vi "Build Profile Steps Commands.vi"(8 "error in":errorcluster, 11 "Profile Steps":string[][](array[string])) -> (0 "error out":errorcluster, 2 "Param Only Commands":T1[](array[typedef]), 3 "Profile Steps Commands":T1[](array[typedef]))   [LabVIEW 2018, in "F4T.lvlib" / "F4T.lvclass"]
doc: "This VI takes a 2D string array containing the temperature chamber profiles steps and outputs the corresponding commands needed for setting the profile to the temperature chamber."
uses:
  F4T.lvclass
  Custom Controls/Command Data.ctl
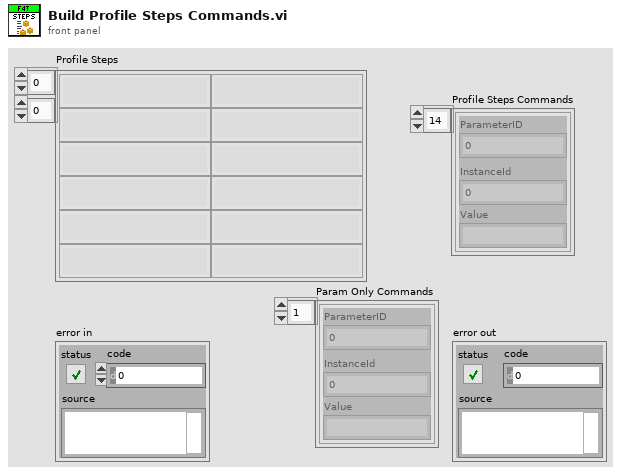
[diagram p1: front panel]
types:
  T1 = typedef "F4T.lvlib/F4T.lvclass/Command Data.ctl" = cluster{"ParameterID":u32, "InstanceId":u32, "Value":string}
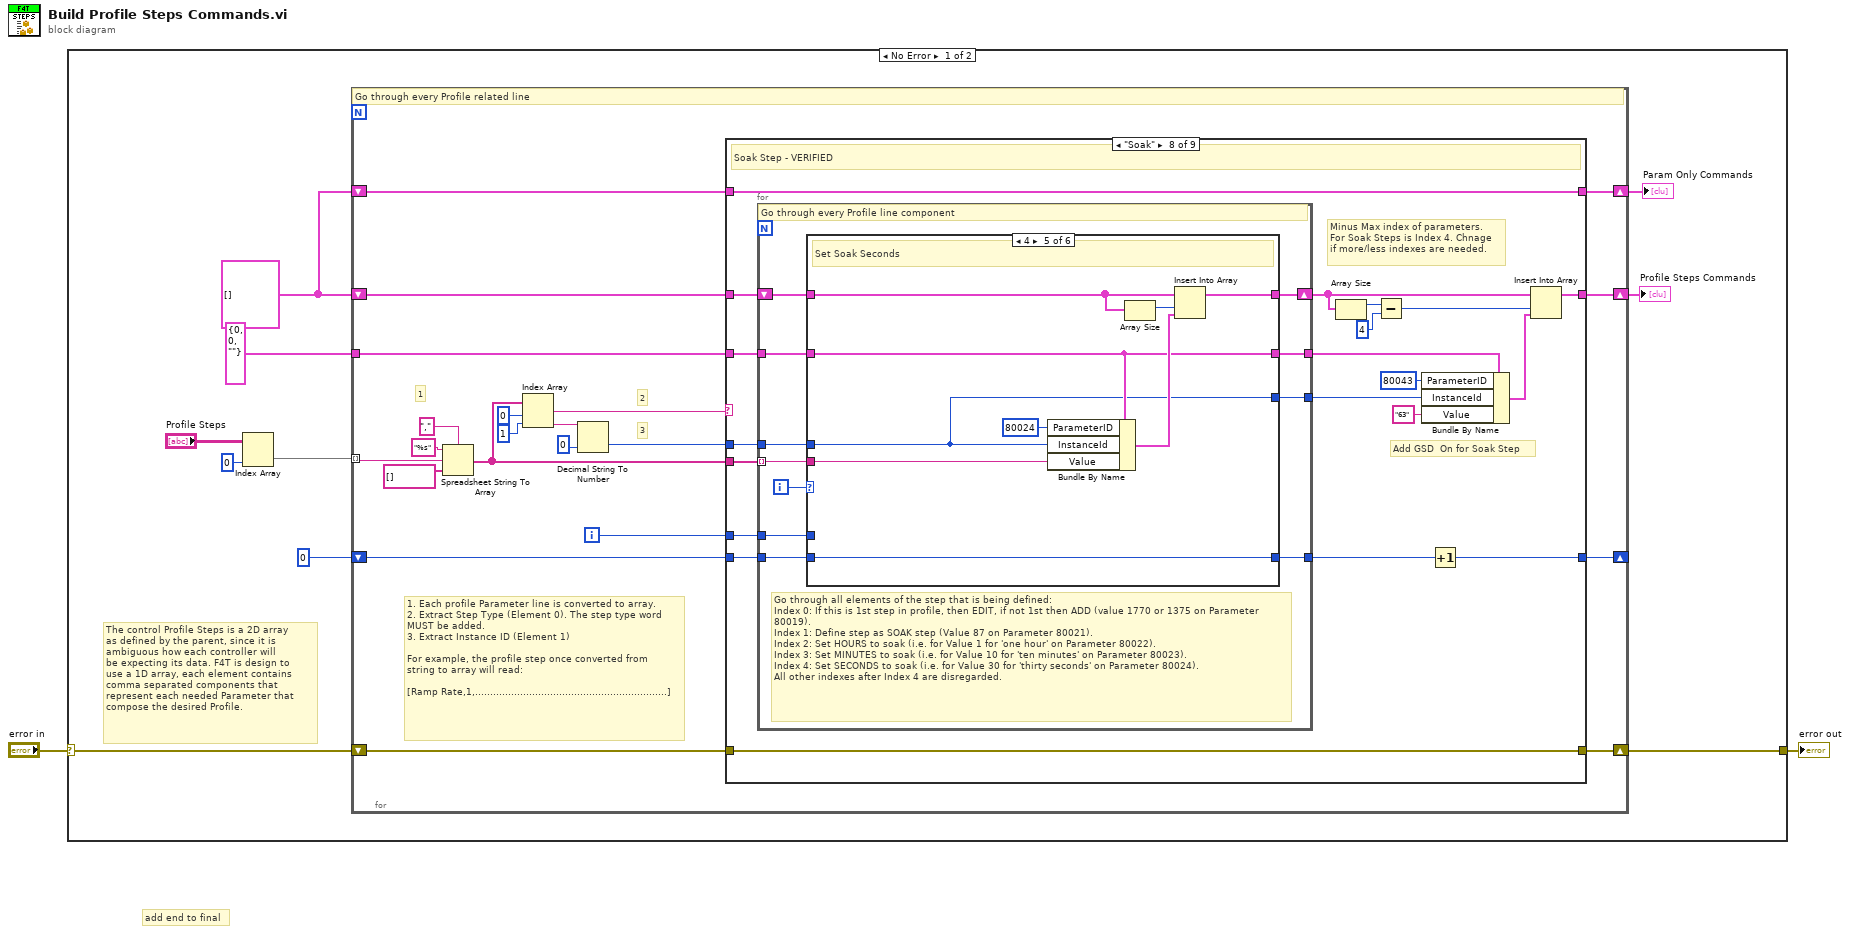
[diagram p0: block diagram]
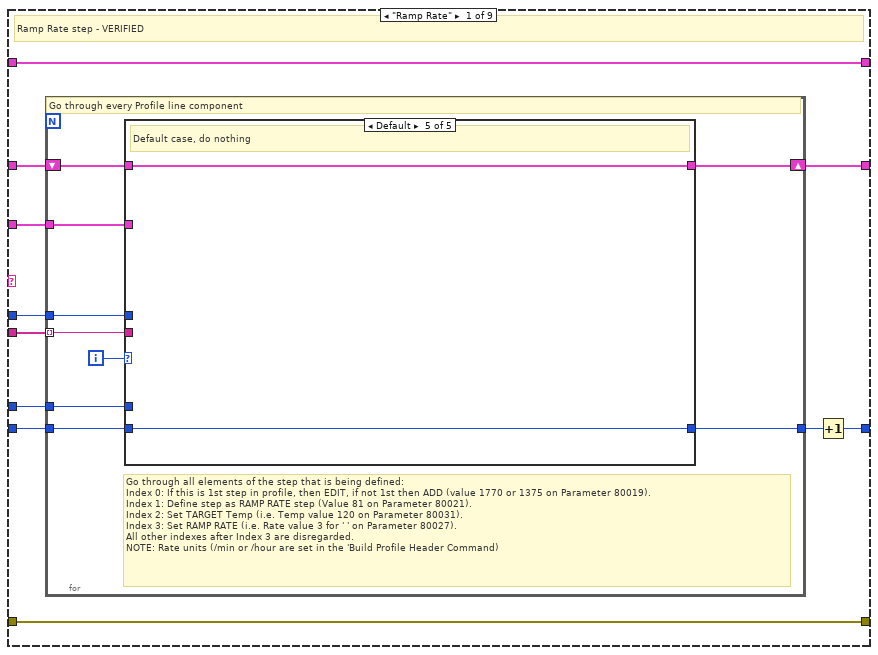
[diagram p2: hidden frame]
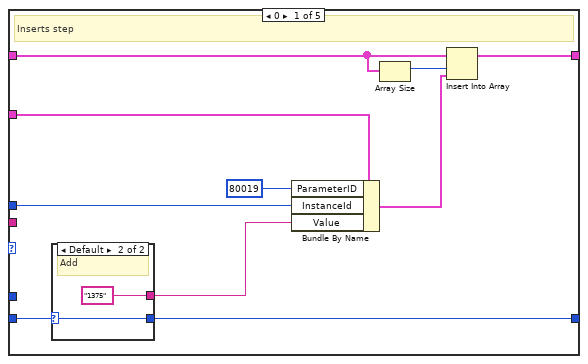
[diagram p3: hidden frame]
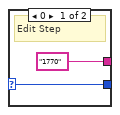
[diagram p4: hidden frame]
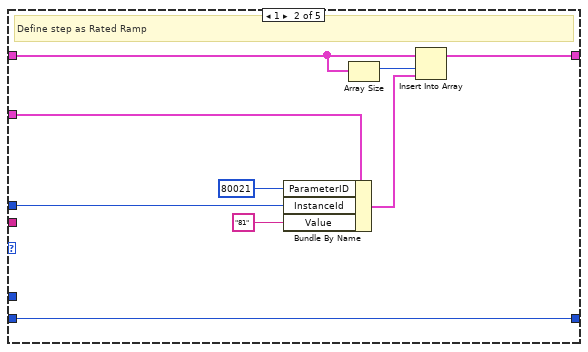
[diagram p5: hidden frame]
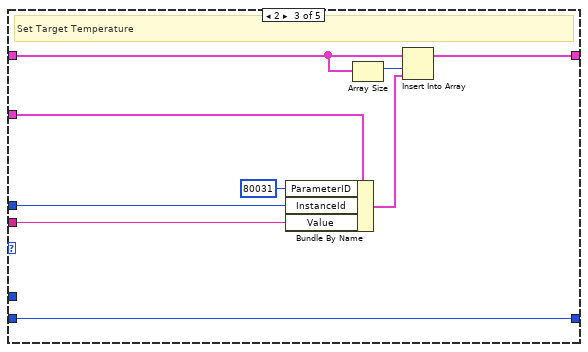
[diagram p6: hidden frame]
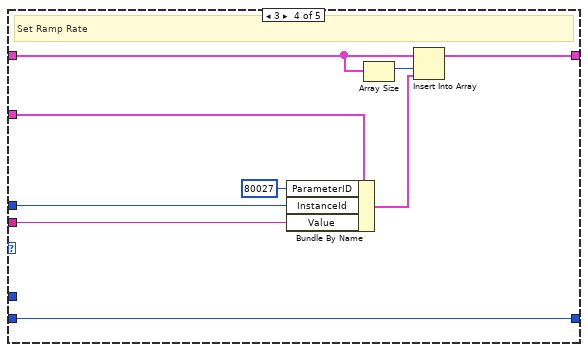
[diagram p7: hidden frame]
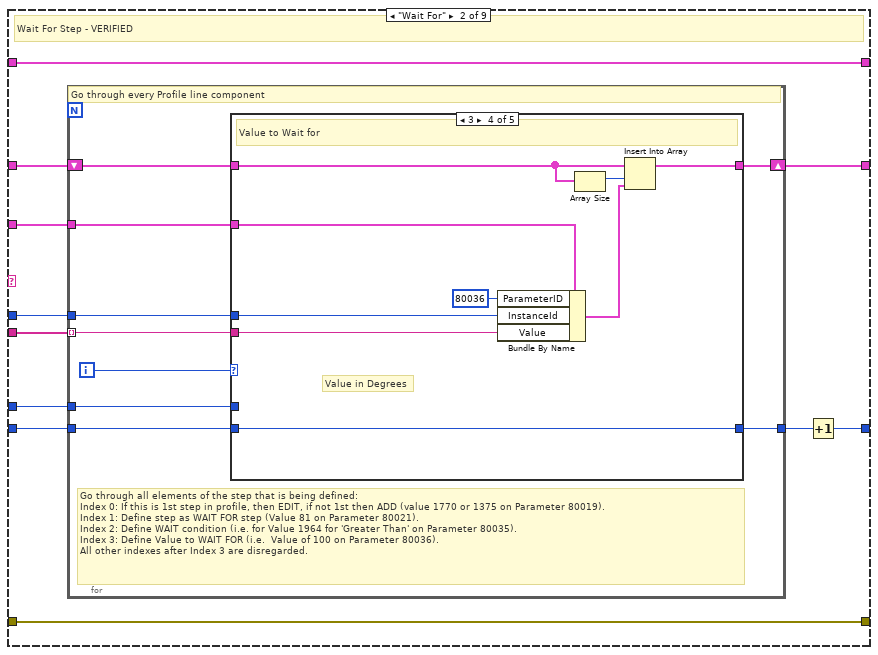
[diagram p8: hidden frame]
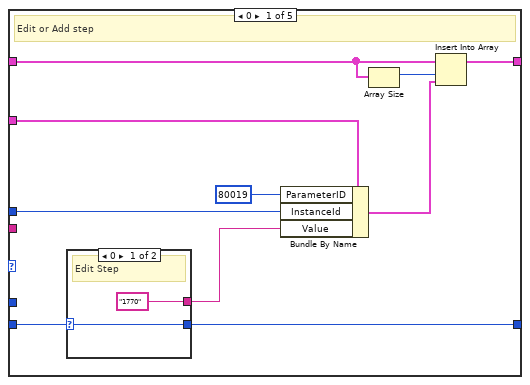
[diagram p9: hidden frame]
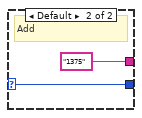
[diagram p10: hidden frame]
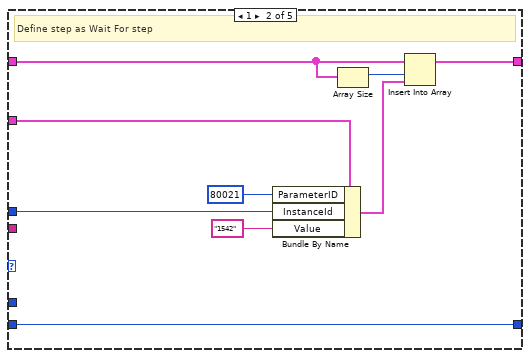
[diagram p11: hidden frame]
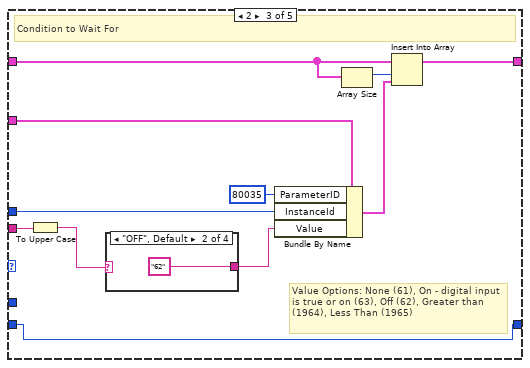
[diagram p12: hidden frame]
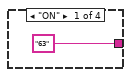
[diagram p13: hidden frame]
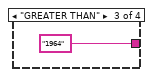
[diagram p14: hidden frame]
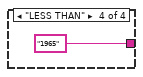
[diagram p15: hidden frame]
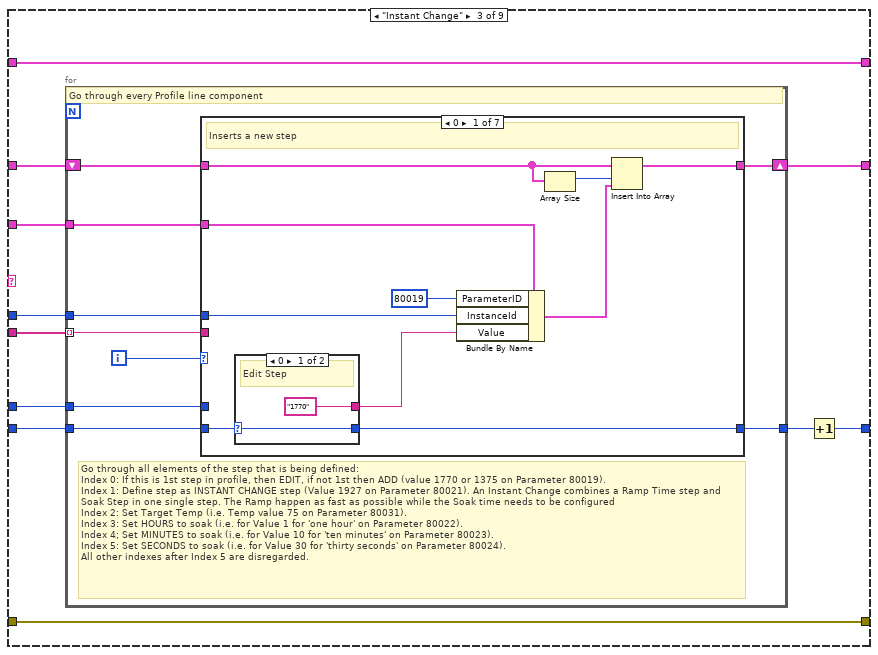
[diagram p17: hidden frame]
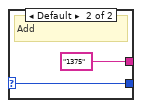
[diagram p18: hidden frame]
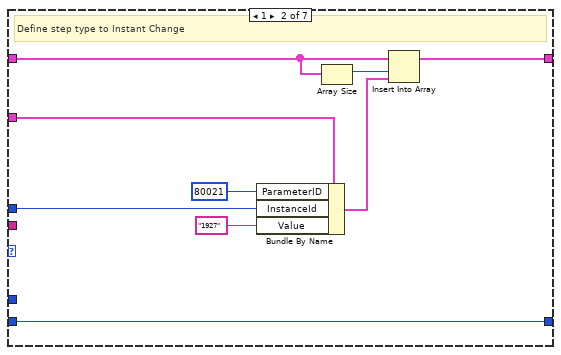
[diagram p19: hidden frame]
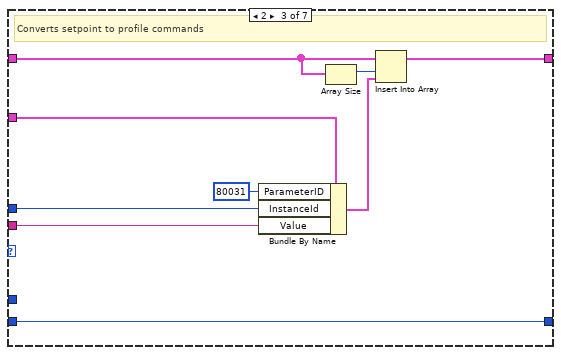
[diagram p20: hidden frame]
diagram:
  # "add end to final"
  n1 = case shown="No Error" "error in" {
    selector: "error in" -> [w11 w555]
    tunnel: [w10 w555] -> w1
    frame No Error {
      w5 = T1[] []
      # "The control Profile Steps is a 2D array\nas defined by the parent, since it is \nambiguous how each controller will\nbe expecting its data. F4T is design to\nuse a 1D array, each element contains\ncomma separated components that\nrepresent each needed Parameter that\ncompose the desired Profile."
      n2 = Index Array(array="Profile Steps", index (col)=0 ("disabled index (col)")) -> (element=w6:string[])  [unwired: 1 in]
      n3 = for {
        tunnel: w6 -> [w25] mode=indexing
        shift-right: [w19] -> w10
        shift-left: w11 -> [w18]
        shift-right: [w29] -> w12
        shift-left: w5 -> [w31]
        tunnel: T1 {"ParameterID"=0, "InstanceId"=0, "Value"=""} ("Command Data") -> [w30]
        shift-right: [w15] -> w4
        shift-left: w5 -> [w16]
        shift-right: [w13] -> _
        shift-left: 0 -> [w14]
        i -> [w17]
        # "3"
        # "1. Each profile Parameter line is converted to array. \n2. Extract Step Type (Element 0). The step type word\nMUST be added.\n3. Extract Instance ID (Element 1)\n\nFor example, the profile step once converted from\nstring to array will read:\n\n[Ramp Rate,1,................................................................]"
        # "1"
        # "2"
        # "Go through every Profile related line"
        n4 = Spreadsheet String To Array(delimiter (Tab)=",", format string="%s", spreadsheet string=w25, array type (2D Dbl)=string[] []) -> (array=w24:string[])
        n5 = Index Array(array=w24, index #1=0 ("index"), index #2=1 ("index")) -> (element #1=w32:string, element #2=w21:string)
        n6 = Decimal String To Number(string=w21, default (0L)=u32 0 ("default (0 I32)")) -> (number=w20:u32)  [unwired: 1 in, 1 out]
        n7 = case shown="\"Soak\"" w32 {
          tunnel: w24 -> [w43 w106 w175 w252 w322 w375 _ w469 w549]
          tunnel: w31 -> [w44 w107 w176 w257 w327 w376 w450 w470 w540]
          tunnel: w30 -> [w42 w105 w174 w256 w326 w374 _ w468 w554]
          tunnel: [w41 w104 w173 w255 w319 w373 w450 w464 w540] -> w29
          tunnel: w20 -> [w40 w103 w172 w253 w323 w372 _ w467 w550]
          tunnel: [w39 w102 w171 w254 w325 w371 w449 w466 w553] -> w19
          tunnel: w18 -> [w39 w102 w171 w254 w325 w371 w449 w466 w553]
          tunnel: w17 -> [w38 w101 w170 w251 w324 w370 _ w465 _]
          tunnel: w16 -> [w37 w100 w169 w250 w313 w369 w448 w454 w542]
          tunnel: [w37 w100 w169 w250 w313 w369 w448 w454 w541] -> w15
          tunnel: w14 -> [w36 w99 w168 w249 w312 w368 w447 w453 w537]
          tunnel: [w34 w97 w166 w247 w310 w366 w447 w451 w536] -> w13
          frame "Ramp Rate" {
            # "Ramp Rate step - VERIFIED"
            n8 = for {
              tunnel: w43 -> [w50] mode=indexing
              tunnel: w40 -> [w49]
              shift-right: [w53] -> w41
              shift-left: w44 -> [w51]
              tunnel: w42 -> [w48]
              tunnel: w38 -> [w47]
              tunnel: w36 -> [w46]
              tunnel: [w45] -> w35
              i -> [w52]
              # "Go through all elements of the step that is being defined:\nIndex 0: If this is 1st step in profile, then EDIT, if not 1st then ADD (value 1770 or 1375 on Parameter 80019).\nIndex 1: Define step as RAMP RATE step (Value 81 on Parameter 80021).\nIndex 2: Set TARGET Temp (i.e. Temp value 120 on Parameter 80031).\nIndex 3: Set RAMP RATE (i.e. Rate value 3 for ' ' on Parameter 80027).\nAll other indexes after Index 3 are disregarded.\nNOTE: Rate units (/min or /hour are set in the 'Build Profile Header Command)"
              # "Go through every Profile line component"
              n9 = case shown="Default" w52 {
                tunnel: [w59 w70 w85 w94 w96] -> w53
                tunnel: w51 -> [w58 w71 w84 w93 w96]
                tunnel: w50 -> [_ _ w81 w87 _]
                tunnel: w49 -> [w62 w74 w83 w92 _]
                tunnel: w48 -> [w60 w73 w82 w91 _]
                tunnel: w47 -> [_ _ _ _ _]
                tunnel: w46 -> [w55 w68 w77 w86 w95]
                tunnel: [w54 w68 w77 w86 w95] -> w45
                frame 0 {
                  # "Inserts step"
                  n10 = case shown="Default" w55 {
                    selector: w55 -> [w64 w66]
                    tunnel: ["1770" ("Value") "1375" ("Value")] -> w56
                    tunnel: [w64 w66] -> w54
                    frame 0 {
                      # "Edit Step"
                    }
                    frame Default {
                      # "Add"
                    }
                  }
                  n11 = Bundle By Name(cluster=w60, "ParameterID"=u32 80019, "InstanceId"=w62, "Value"=w56) -> (w57:T1)
                  n12 = Array Size(array=w58) -> (size(s)=w61:i32)
                  n13 = Insert Into Array(array=w58, index=w61, new element=w57) -> (w59:T1[])
                }
                frame 1 {
                  # "Define step as Rated Ramp"
                  n14 = Bundle By Name(cluster=w73, "ParameterID"=u32 80021, "InstanceId"=w74, "Value"="81") -> (w69:T1)
                  n15 = Array Size(array=w71) -> (size(s)=w72:i32)
                  n16 = Insert Into Array(array=w71, index=w72, new element=w69) -> (w70:T1[])
                }
                frame 2 {
                  # "Set Target Temperature"
                  n17 = Bundle By Name(cluster=w82, "ParameterID"=u32 80031, "InstanceId"=w83, "Value"=w81) -> (w78:T1)
                  n18 = Array Size(array=w84) -> (size(s)=w79:i32)
                  n19 = Insert Into Array(array=w84, index=w79, new element=w78) -> (w85:T1[])
                }
                frame 3 {
                  # "Set Ramp Rate"
                  n20 = Bundle By Name(cluster=w91, "ParameterID"=u32 80027, "InstanceId"=w92, "Value"=w87) -> (w88:T1)
                  n21 = Array Size(array=w93) -> (size(s)=w89:i32)
                  n22 = Insert Into Array(array=w93, index=w89, new element=w88) -> (w94:T1[])
                }
                frame Default {
                  # "Default case, do nothing"
                }
              }
            }
            n23 = Increment(x=w35) -> (x+1=w34:i32)
          }
          frame "Wait For" {
            # "Wait For Step - VERIFIED"
            n24 = for {
              tunnel: w106 -> [w113] mode=indexing
              tunnel: w103 -> [w112]
              shift-right: [w116] -> w104
              shift-left: w107 -> [w114]
              tunnel: w105 -> [w111]
              tunnel: w101 -> [w110]
              tunnel: w99 -> [w109]
              tunnel: [w108] -> w98
              i -> [w115]
              # "Go through all elements of the step that is being defined:\nIndex 0: If this is 1st step in profile, then EDIT, if not 1st then ADD (value 1770 or 1375 on Parameter 80019).\nIndex 1: Define step as WAIT FOR step (Value 81 on Parameter 80021).\nIndex 2: Define WAIT condition (i.e. for Value 1964 for 'Greater Than' on Parameter 80035).\nIndex 3: Define Value to WAIT FOR (i.e.  Value of 100 on Parameter 80036).\nAll other indexes after Index 3 are disregarded."
              # "Go through every Profile line component"
              n25 = case shown="3" w115 {
                tunnel: [w121 w133 w150 w163 w165] -> w116
                tunnel: w114 -> [w120 w134 w149 w162 w165]
                tunnel: w113 -> [_ _ w143 w156 _]
                tunnel: w112 -> [w124 w137 w148 w161 _]
                tunnel: w111 -> [w122 w136 w147 w160 _]
                tunnel: w110 -> [_ _ _ _ _]
                tunnel: w109 -> [w118 w131 w140 w155 w164]
                tunnel: [w117 w131 w140 w155 w164] -> w108
                frame 0 {
                  # "Edit or Add step"
                  n26 = case shown="0" w118 {
                    selector: w118 -> [w127 w129]
                    tunnel: ["1770" ("Value") "1375" ("Value")] -> w125
                    tunnel: [w127 w129] -> w117
                    frame 0 {
                      # "Edit Step"
                    }
                    frame Default {
                      # "Add"
                    }
                  }
                  n27 = Bundle By Name(cluster=w122, "ParameterID"=u32 80019, "InstanceId"=w124, "Value"=w125) -> (w119:T1)
                  n28 = Array Size(array=w120) -> (size(s)=w123:i32)
                  n29 = Insert Into Array(array=w120, index=w123, new element=w119) -> (w121:T1[])
                }
                frame 1 {
                  # "Define step as Wait For step"
                  n30 = Bundle By Name(cluster=w136, "ParameterID"=u32 80021, "InstanceId"=w137, "Value"="1542") -> (w132:T1)
                  n31 = Array Size(array=w134) -> (size(s)=w135:i32)
                  n32 = Insert Into Array(array=w134, index=w135, new element=w132) -> (w133:T1[])
                }
                frame 2 {
                  # "Value Options: None (61), On - digital input is true or on (63), Off (62), Greater than (1964), Less Than (1965)"
                  # "Condition to Wait For"
                  n33 = To Upper Case(1:w143) -> (0:w142:string)
                  n34 = case shown="\"OFF\", Default" w142 {
                    tunnel: ["63" ("Value") "62" ("Value") "1964" ("Value") "1965" ("Value")] -> w141
                    frame "ON" {
                    }
                    frame "OFF", Default {
                    }
                    frame "GREATER THAN" {
                    }
                    frame "LESS THAN" {
                    }
                  }
                  n35 = Bundle By Name(cluster=w147, "ParameterID"=u32 80035, "InstanceId"=w148, "Value"=w141) -> (w144:T1)
                  n36 = Array Size(array=w149) -> (size(s)=w145:i32)
                  n37 = Insert Into Array(array=w149, index=w145, new element=w144) -> (w150:T1[])
                }
                frame 3 {
                  # "Value in Degrees"
                  # "Value to Wait for"
                  n38 = Bundle By Name(cluster=w160, "ParameterID"=u32 80036, "InstanceId"=w161, "Value"=w156) -> (w157:T1)
                  n39 = Array Size(array=w162) -> (size(s)=w158:i32)
                  n40 = Insert Into Array(array=w162, index=w158, new element=w157) -> (w163:T1[])
                }
                frame Default {
                  # "Defualt case, do nothing"
                }
              }
            }
            n41 = Increment(x=w98) -> (x+1=w97:i32)
          }
          frame "Instant Change" {
            n42 = for {
              tunnel: w175 -> [w182] mode=indexing
              tunnel: w172 -> [w181]
              shift-right: [w185] -> w173
              shift-left: w176 -> [w183]
              tunnel: w174 -> [w180]
              tunnel: w170 -> [w179]
              tunnel: w168 -> [w178]
              tunnel: [w177] -> w167
              i -> [w184]
              # "Go through all elements of the step that is being defined:\nIndex 0: If this is 1st step in profile, then EDIT, if not 1st then ADD (value 1770 or 1375 on Parameter 80019).\nIndex 1: Define step as INSTANT CHANGE step (Value 1927 on Parameter 80021). An Instant Change combines a Ramp Time step and Soak Step in one single step. The Ramp happen as fast as possible while the Soak time needs to be configured\nIndex 2: Set Target Temp (i.e. Temp value 75 on Parameter 80031).\nIndex 3: Set HOURS to soak (i.e. for Value 1 for 'one hour' on Parameter 80022).\nIndex 4; Set MINUTES to soak (i.e. for Value 10 for 'ten minutes' on Parameter 80023).\nIndex 5: Set SECONDS to soak (i.e. for Value 30 for 'thirty seconds' on Parameter 80024).\nAll other indexes after Index 5 are disregarded."
              # "Go through every Profile line component"
              n43 = case shown="0" w184 {
                tunnel: [w191 w202 w217 w226 w235 w244 w246] -> w185
                tunnel: w183 -> [w190 w203 w216 w225 w234 w243 w246]
                tunnel: w182 -> [_ _ w213 w222 w231 w240 _]
                tunnel: w181 -> [w194 w206 w215 w224 w233 w242 _]
                tunnel: w180 -> [w192 w205 w214 w223 w232 w241 _]
                tunnel: w179 -> [_ _ _ _ _ _ _]
                tunnel: w178 -> [w187 w200 w209 w218 w227 w236 w245]
                tunnel: [w186 w200 w209 w218 w227 w236 w245] -> w177
                frame 0 {
                  # "Inserts a new step"
                  n44 = case shown="0" w187 {
                    selector: w187 -> [w196 w198]
                    tunnel: ["1770" ("Value") "1375" ("Value")] -> w188
                    tunnel: [w196 w198] -> w186
                    frame 0 {
                      # "Edit Step"
                    }
                    frame Default {
                      # "Add"
                    }
                  }
                  n45 = Bundle By Name(cluster=w192, "ParameterID"=u32 80019, "InstanceId"=w194, "Value"=w188) -> (w189:T1)
                  n46 = Array Size(array=w190) -> (size(s)=w193:i32)
                  n47 = Insert Into Array(array=w190, index=w193, new element=w189) -> (w191:T1[])
                }
                frame 1 {
                  # "Define step type to Instant Change"
                  n48 = Bundle By Name(cluster=w205, "ParameterID"=u32 80021, "InstanceId"=w206, "Value"="1927") -> (w201:T1)
                  n49 = Array Size(array=w203) -> (size(s)=w204:i32)
                  n50 = Insert Into Array(array=w203, index=w204, new element=w201) -> (w202:T1[])
                }
                frame 2 {
                  # "Converts setpoint to profile commands"
                  n51 = Bundle By Name(cluster=w214, "ParameterID"=u32 80031, "InstanceId"=w215, "Value"=w213) -> (w210:T1)
                  n52 = Array Size(array=w216) -> (size(s)=w211:i32)
                  n53 = Insert Into Array(array=w216, index=w211, new element=w210) -> (w217:T1[])
                }
                frame 3 {
                  # "Set Soak hours"
                  n54 = Bundle By Name(cluster=w223, "ParameterID"=u32 80022, "InstanceId"=w224, "Value"=w222) -> (w219:T1)
                  n55 = Array Size(array=w225) -> (size(s)=w220:i32)
                  n56 = Insert Into Array(array=w225, index=w220, new element=w219) -> (w226:T1[])
                }
                frame 4 {
                  # "Set Soak minutes"
                  n57 = Bundle By Name(cluster=w232, "ParameterID"=u32 80023, "InstanceId"=w233, "Value"=w231) -> (w228:T1)
                  n58 = Array Size(array=w234) -> (size(s)=w229:i32)
                  n59 = Insert Into Array(array=w234, index=w229, new element=w228) -> (w235:T1[])
                }
                frame 5 {
                  # "Set Soak seconds"
                  n60 = Bundle By Name(cluster=w241, "ParameterID"=u32 80024, "InstanceId"=w242, "Value"=w240) -> (w237:T1)
                  n61 = Array Size(array=w243) -> (size(s)=w238:i32)
                  n62 = Insert Into Array(array=w243, index=w238, new element=w237) -> (w244:T1[])
                }
                frame Default {
                  # "Default case, do nothing"
                }
              }
            }
            n63 = Increment(x=w167) -> (x+1=w166:i32)
          }
          frame "Jump" {
            # "Jump Step VERIFIED"
            n64 = for {
              tunnel: w252 -> [w263] mode=indexing
              tunnel: w253 -> [w262]
              shift-right: [w266] -> w255
              shift-left: w257 -> [w264]
              tunnel: w256 -> [w261]
              tunnel: w251 -> [w260]
              tunnel: w249 -> [w259]
              tunnel: [w258] -> w248
              i -> [w265]
              # "Go through all elements of the step that is being defined:\nIndex 0: If this is 1st step in profile, then EDIT, if not 1st then ADD (value 1770 or 1375 on Parameter 80019).\nIndex 1: Define step as JUMP step (Value 116 on Parameter 80021).\nIndex 2: Define the previous step to jump to (i.e. 1 for Step 1 on Parameter 80025).\nIndex 3: Define Jump COUNT (i.e. 5 for 5 iterations on Parameter 80026).\nAll other indexes after Index 3 are disregarded."
              # "Go through every Profile line component"
              n65 = case shown="0" w265 {
                tunnel: [w272 w283 w298 w307 w309] -> w266
                tunnel: w264 -> [w271 w284 w297 w306 w309]
                tunnel: w263 -> [_ _ w291 w300 _]
                tunnel: w262 -> [w275 w287 w296 w305 _]
                tunnel: w261 -> [w273 w286 w295 w304 _]
                tunnel: w260 -> [_ _ _ _ _]
                tunnel: w259 -> [w268 w281 w290 w299 w308]
                tunnel: [w267 w281 w290 w299 w308] -> w258
                frame 0 {
                  # "Inserts a new step"
                  n66 = case shown="0" w268 {
                    selector: w268 -> [w277 w279]
                    tunnel: ["1770" ("Value") "1375" ("Value")] -> w269
                    tunnel: [w277 w279] -> w267
                    frame 0 {
                      # "Edit Step"
                    }
                    frame Default {
                      # "Add"
                    }
                  }
                  n67 = Bundle By Name(cluster=w273, "ParameterID"=u32 80019, "InstanceId"=w275, "Value"=w269) -> (w270:T1)
                  n68 = Array Size(array=w271) -> (size(s)=w274:i32)
                  n69 = Insert Into Array(array=w271, index=w274, new element=w270) -> (w272:T1[])
                }
                frame 1 {
                  # "Define step type to Jump"
                  n70 = Bundle By Name(cluster=w286, "ParameterID"=u32 80021, "InstanceId"=w287, "Value"="116") -> (w282:T1)
                  n71 = Array Size(array=w284) -> (size(s)=w285:i32)
                  n72 = Insert Into Array(array=w284, index=w285, new element=w282) -> (w283:T1[])
                }
                frame 2 {
                  # "Converts setpoint to profile commands"
                  n73 = Bundle By Name(cluster=w295, "ParameterID"=u32 80025, "InstanceId"=w296, "Value"=w291) -> (w292:T1)
                  n74 = Array Size(array=w297) -> (size(s)=w293:i32)
                  n75 = Insert Into Array(array=w297, index=w293, new element=w292) -> (w298:T1[])
                }
                frame 3 {
                  # "Converts setpoint to profile commands"
                  n76 = Bundle By Name(cluster=w304, "ParameterID"=u32 80026, "InstanceId"=w305, "Value"=w300) -> (w301:T1)
                  n77 = Array Size(array=w306) -> (size(s)=w302:i32)
                  n78 = Insert Into Array(array=w306, index=w302, new element=w301) -> (w307:T1[])
                }
                frame Default {
                  # "Default case, do nothing"
                }
              }
            }
            n79 = Increment(x=w248) -> (x+1=w247:i32)
          }
          frame "End" {
            # "Set CONTROL LOOP END STATE \n(i.e. Value 100 for 'User' on \nParameter 80073)."
            # "End step - VERIFIED"
            n80 = for {
              tunnel: w322 -> [w335] mode=indexing
              tunnel: w323 -> [w334]
              shift-right: [w338] -> w320
              shift-left: w327 -> [w336]
              tunnel: w326 -> [w333]
              tunnel: w324 -> [w332]
              tunnel: [w331] -> w316
              tunnel: [w330] -> w317
              tunnel: w312 -> [w329]
              tunnel: [w328] -> w311
              i -> [w337]
              # "Go through all elements of the step that is being defined:\nIndex 0: If this is 1st step in profile, then EDIT, if not 1st then ADD (value 1770 or 1375 on Parameter 80019).\nIndex 1: Define step as END step (Value 27 on Parameter 80021).\nAll other indexes after Index 2 are disregarded."
              # "Go through every Profile line component"
              n81 = case shown="0" w337 {
                tunnel: [w346 w357 w365] -> w338
                tunnel: w336 -> [w345 w358 w365]
                tunnel: w335 -> [_ _ _]
                tunnel: w334 -> [w341 w354 w363]
                tunnel: w333 -> [w342 w355 w364]
                tunnel: w332 -> [_ _ _]
                tunnel: [w342 w355 w364] -> w331
                tunnel: [w341 w354 w363] -> w330
                tunnel: w329 -> [w340 w353 w362]
                tunnel: [w339 w353 w362] -> w328
                frame 0 {
                  # "Inserts a new step"
                  n82 = case shown="0" w340 {
                    selector: w340 -> [w349 w351]
                    tunnel: ["1770" ("Value") "1375" ("Value")] -> w343
                    tunnel: [w349 w351] -> w339
                    frame 0 {
                      # "Edit Step"
                    }
                    frame Default {
                      # "Add"
                    }
                  }
                  n83 = Bundle By Name(cluster=w342, "ParameterID"=u32 80019, "InstanceId"=w341, "Value"=w343) -> (w344:T1)
                  n84 = Array Size(array=w345) -> (size(s)=w347:i32)
                  n85 = Insert Into Array(array=w345, index=w347, new element=w344) -> (w346:T1[])
                }
                frame 1 {
                  # "Define step type to End"
                  n86 = Bundle By Name(cluster=w355, "ParameterID"=u32 80021, "InstanceId"=w354, "Value"="27") -> (w356:T1)
                  n87 = Array Size(array=w358) -> (size(s)=w359:i32)
                  n88 = Insert Into Array(array=w358, index=w359, new element=w356) -> (w357:T1[])
                }
                frame Default {
                  # "Default case, do nothing"
                }
              }
            }
            n89 = Array Size(array=w320) -> (size(s)=w321:i32)
            n90 = Bundle By Name(cluster=w316, "ParameterID"=u32 80073, "InstanceId"=w317, "Value"="100") -> (w315:T1)
            n91 = Increment(x=w311) -> (x+1=w310:i32)
            n92 = Insert Into Array(array=w320, index=w321, new element=w315) -> (w319:T1[])
          }
          frame "Ramp Time" {
            # "Ramp Time step - VERIFIED"
            n93 = for {
              tunnel: w375 -> [w382] mode=indexing
              tunnel: w372 -> [w381]
              shift-right: [w385] -> w373
              shift-left: w376 -> [w383]
              tunnel: w374 -> [w380]
              tunnel: w370 -> [w379]
              tunnel: w368 -> [w378]
              tunnel: [w377] -> w367
              i -> [w384]
              # "Go through all elements of the step that is being defined:\nIndex 0: If this is 1st step in profile, then EDIT, if not 1st then ADD (value 1770 or 1375 on Parameter 80019).\nIndex 1: Define step as RAMP TIME step (Value 1928 on Parameter 80021). \nIndex 2: Set Target Temp (i.e. Temp value 75 on Parameter 80031).\nIndex 3: Set HOURS to soak (i.e. for Value 1 for 'one hour' on Parameter 80022).\nIndex 4; Set MINUTES to soak (i.e. for Value 10 for 'ten minutes' on Parameter 80023).\nIndex 5: Set SECONDS to soak (i.e. for Value 30 for 'thirty seconds' on Parameter 80024).\nAll other indexes after Index 5 are disregarded."
              # "Go through every Profile line component"
              n94 = case shown="0" w384 {
                tunnel: [w391 w402 w417 w426 w435 w444 w446] -> w385
                tunnel: w383 -> [w390 w403 w416 w425 w434 w443 w446]
                tunnel: w382 -> [_ _ w410 w419 w428 w437 _]
                tunnel: w381 -> [w394 w406 w415 w424 w433 w442 _]
                tunnel: w380 -> [w392 w405 w414 w423 w432 w441 _]
                tunnel: w379 -> [_ _ _ _ _ _ _]
                tunnel: w378 -> [w387 w400 w409 w418 w427 w436 w445]
                tunnel: [w386 w400 w409 w418 w427 w436 w445] -> w377
                frame 0 {
                  # "Inserts step"
                  n95 = case shown="0" w387 {
                    selector: w387 -> [w396 w398]
                    tunnel: ["1770" ("Value") "1375" ("Value")] -> w388
                    tunnel: [w396 w398] -> w386
                    frame 0 {
                      # "Edit Step"
                    }
                    frame Default {
                      # "Add"
                    }
                  }
                  n96 = Bundle By Name(cluster=w392, "ParameterID"=u32 80019, "InstanceId"=w394, "Value"=w388) -> (w389:T1)
                  n97 = Array Size(array=w390) -> (size(s)=w393:i32)
                  n98 = Insert Into Array(array=w390, index=w393, new element=w389) -> (w391:T1[])
                }
                frame 1 {
                  # "Define step type to a Timed Ramp"
                  n99 = Bundle By Name(cluster=w405, "ParameterID"=u32 80021, "InstanceId"=w406, "Value"="1928") -> (w401:T1)
                  n100 = Array Size(array=w403) -> (size(s)=w404:i32)
                  n101 = Insert Into Array(array=w403, index=w404, new element=w401) -> (w402:T1[])
                }
                frame 2 {
                  # "Set Target Temperature"
                  n102 = Bundle By Name(cluster=w414, "ParameterID"=u32 80031, "InstanceId"=w415, "Value"=w410) -> (w411:T1)
                  n103 = Array Size(array=w416) -> (size(s)=w412:i32)
                  n104 = Insert Into Array(array=w416, index=w412, new element=w411) -> (w417:T1[])
                }
                frame 3 {
                  # "Set Target Temperature"
                  n105 = Bundle By Name(cluster=w423, "ParameterID"=u32 80022, "InstanceId"=w424, "Value"=w419) -> (w420:T1)
                  n106 = Array Size(array=w425) -> (size(s)=w421:i32)
                  n107 = Insert Into Array(array=w425, index=w421, new element=w420) -> (w426:T1[])
                }
                frame 4 {
                  # "Set Target Temperature"
                  n108 = Bundle By Name(cluster=w432, "ParameterID"=u32 80023, "InstanceId"=w433, "Value"=w428) -> (w429:T1)
                  n109 = Array Size(array=w434) -> (size(s)=w430:i32)
                  n110 = Insert Into Array(array=w434, index=w430, new element=w429) -> (w435:T1[])
                }
                frame 5 {
                  # "Set Target Temperature"
                  n111 = Bundle By Name(cluster=w441, "ParameterID"=u32 80024, "InstanceId"=w442, "Value"=w437) -> (w438:T1)
                  n112 = Array Size(array=w443) -> (size(s)=w439:i32)
                  n113 = Insert Into Array(array=w443, index=w439, new element=w438) -> (w444:T1[])
                }
                frame Default {
                  # "Converts setpoint to profile commands"
                }
              }
            }
            n114 = Increment(x=w367) -> (x+1=w366:i32)
          }
          frame Default {
          }
          frame "Soak" {
            # "Minus Max index of parameters.\nFor Soak Steps is Index 4. Chnage\nif more/less indexes are needed."
            # "Add GSD  On for Soak Step"
            # "Soak Step - VERIFIED"
            n115 = for {
              tunnel: w469 -> [w478] mode=indexing
              tunnel: w467 -> [w477]
              shift-right: [w481] -> w458
              shift-left: w470 -> [w479]
              tunnel: w468 -> [w476]
              tunnel: w465 -> [w475]
              tunnel: [w474] -> w462
              tunnel: [w473] -> w459
              tunnel: w453 -> [w472]
              tunnel: [w471] -> w452
              i -> [w480]
              # "Go through all elements of the step that is being defined:\nIndex 0: If this is 1st step in profile, then EDIT, if not 1st then ADD (value 1770 or 1375 on Parameter 80019).\nIndex 1: Define step as SOAK step (Value 87 on Parameter 80021).\nIndex 2: Set HOURS to soak (i.e. for Value 1 for 'one hour' on Parameter 80022).\nIndex 3: Set MINUTES to soak (i.e. for Value 10 for 'ten minutes' on Parameter 80023).\nIndex 4: Set SECONDS to soak (i.e. for Value 30 for 'thirty seconds' on Parameter 80024).\nAll other indexes after Index 4 are disregarded."
              # "Go through every Profile line component"
              n116 = case shown="4" w480 {
                tunnel: [w489 w500 w513 w522 w531 w535] -> w481
                tunnel: w479 -> [w488 w501 w512 w521 w530 w535]
                tunnel: w478 -> [_ _ w511 w520 w529 _]
                tunnel: w477 -> [w484 w498 w506 w515 w524 w533]
                tunnel: w476 -> [w485 w497 w507 w516 w525 w534]
                tunnel: w475 -> [_ _ _ _ _ _]
                tunnel: [w485 w497 w507 w516 w525 w534] -> w474
                tunnel: [w484 w498 w506 w515 w524 w533] -> w473
                tunnel: w472 -> [w483 w496 w505 w514 w523 w532]
                tunnel: [w482 w496 w505 w514 w523 w532] -> w471
                frame 0 {
                  # "Edit or Add step"
                  n117 = case shown="Default" w483 {
                    selector: w483 -> [w492 w494]
                    tunnel: ["1770" ("Value") "1375" ("Value")] -> w486
                    tunnel: [w492 w494] -> w482
                    frame 0 {
                      # "Edit Step"
                    }
                    frame Default {
                      # "Add"
                    }
                  }
                  n118 = Bundle By Name(cluster=w485, "ParameterID"=u32 80019, "InstanceId"=w484, "Value"=w486) -> (w487:T1)
                  n119 = Array Size(array=w488) -> (size(s)=w490:i32)
                  n120 = Insert Into Array(array=w488, index=w490, new element=w487) -> (w489:T1[])
                }
                frame 1 {
                  # "Define step type to Soak"
                  n121 = Bundle By Name(cluster=w497, "ParameterID"=u32 80021, "InstanceId"=w498, "Value"="87") -> (w499:T1)
                  n122 = Array Size(array=w501) -> (size(s)=w502:i32)
                  n123 = Insert Into Array(array=w501, index=w502, new element=w499) -> (w500:T1[])
                }
                frame 2 {
                  # "Set Soak Hours"
                  n124 = Bundle By Name(cluster=w507, "ParameterID"=u32 80022, "InstanceId"=w506, "Value"=w511) -> (w508:T1)
                  n125 = Array Size(array=w512) -> (size(s)=w509:i32)
                  n126 = Insert Into Array(array=w512, index=w509, new element=w508) -> (w513:T1[])
                }
                frame 3 {
                  # "Set Soak Minutes"
                  n127 = Bundle By Name(cluster=w516, "ParameterID"=u32 80023, "InstanceId"=w515, "Value"=w520) -> (w517:T1)
                  n128 = Array Size(array=w521) -> (size(s)=w518:i32)
                  n129 = Insert Into Array(array=w521, index=w518, new element=w517) -> (w522:T1[])
                }
                frame 4 {
                  # "Set Soak Seconds"
                  n130 = Bundle By Name(cluster=w525, "ParameterID"=u32 80024, "InstanceId"=w524, "Value"=w529) -> (w526:T1)
                  n131 = Array Size(array=w530) -> (size(s)=w527:i32)
                  n132 = Insert Into Array(array=w530, index=w527, new element=w526) -> (w531:T1[])
                }
                frame Default {
                  # "Default case, do nothing"
                }
              }
            }
            n133 = Array Size(array=w458) -> (size(s)=w457:i32)
            n134 = Subtract(x=w457, y=4) -> (x-y=w456:i32)
            n135 = Bundle By Name(cluster=w462, "ParameterID"=u32 80043, "InstanceId"=w459, "Value"="63") -> (w460:T1)
            n136 = Increment(x=w452) -> (x+1=w451:i32)
            n137 = Insert Into Array(array=w458, index=w456, new element=w460) -> (w464:T1[])
          }
          frame "Parameter" {
            # "The Parameter case is used to send any particular command that is not particularly tied to a running step.\nSend this parameter command in the following string convention:\nParameter (this is literally the word Parameter), InstanceId, ParameterID, Value."
            # "Case dedicated for single parameter processing"
            n138 = Index Array(array=w549, index #1=2 ("index"), index #2=3 ("index")) -> (element #1=w545:string, element #2=w546:string)
            n139 = Equal To 0?(x=w537) -> (x = 0?=w539:bool)
            n140 = Decimal String To Number(string=w545, default (0L)=u32 0) -> (number=w544:u32)  [unwired: 1 in, 1 out]
            n141 = Bundle By Name(cluster=w554, "ParameterID"=w544, "InstanceId"=w550, "Value"=w546) -> (w551:T1)
            n142 = Select(t=0, s=w539, f=w537) -> (s? t:f=w536:i32)
            n143 = Array Size(array=w542) -> (size(s)=w552:i32)
            n144 = Insert Into Array(array=w542, index=w552, new element=w551) -> (w541:T1[])
          }
        }
      }
      "Profile Steps Commands" <- w12
      "Param Only Commands" <- w4
    }
    frame Error {
    }
  }
  "error out" <- w1
